vi "9759 RevB Read.vi"(5 "FIFO Indexes.Read":T3, 6 "Device Outputs in":dbl[](array[numeric]), 7 "Settings.PositionCals":T2(array[cluster]), 8 "error in":errorcluster, 9 "dt (sec)":sgl, 11 "FPGA Ref in":T4) -> (0 "error out":errorcluster, 2 "Data":T1, 3 "FPGA Ref out":T4, 4 "Device Outputs out":dbl[](array[numeric]))   [LabVIEW 2015, in "NI 9759 RevB Custom Device.lvlib"]
uses:
  NI 9759 RevB Custom Device.lvlib
  Shared/Types/9759 RevB FPGA Ref.ctl
  <vilib>/Utility/error.llb/Error Cluster From Error Code.vi
  <vilib>/rvi/errors/niLvFpgaAdjustHostInterfaceError.vi
  <vilib>/rvi/interface/nirviReadWriteControl/nirviReadWriteControl.xnode
  NiFpgaLv.dll
  <vilib>/rvi/interface/Simulation/niFpgaSimulationCallBeginRW.vi
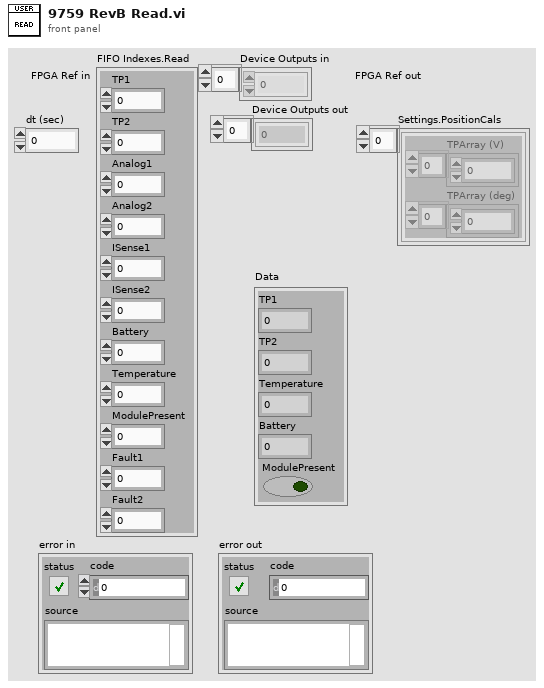
[diagram p1: front panel]
types:
  T1 = cluster{"TP1":sgl, "TP2":sgl, "Temperature":sgl, "Battery":sgl, "ModulePresent":bool}
  T2 = cluster{"TPArray (V)":sgl[], "TPArray (deg)":sgl[]}[]
  T3 = cluster{"TP1":i32, "TP2":i32, "Analog1":i32, "Analog2":i32, "ISense1":i32, "ISense2":i32, "Battery":i32, "Temperature":i32, "ModulePresent":i32, "Fault1":i32, "Fault2":i32}
  T4 = typedef "NI 9759 RevB Custom Device.lvlib/9759 RevB FPGA Ref.ctl" = refnum<k20>
  T5 = cluster{"ModulePresent":bool, "ISense1":i16, "ISense2":i16, "Analog1":i16, "Analog2":i16, "Battery":i16, "Temperature":i16, "Fault1":bool, "Fault2":bool}
  T6 = cluster{"TPArray (V)":sgl[], "TPArray (deg)":sgl[]}
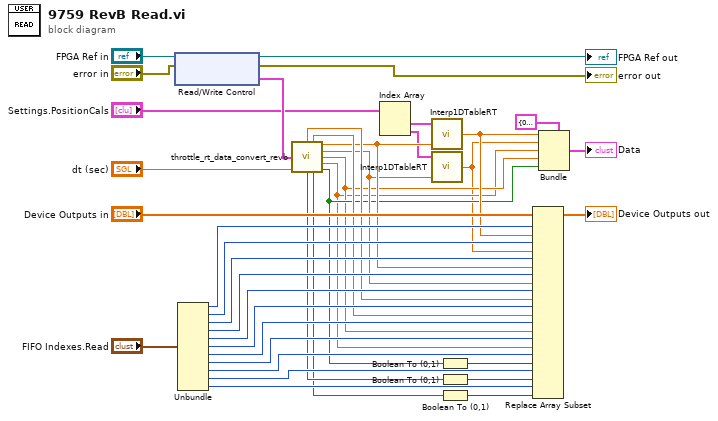
[diagram p0: block diagram]
diagram:
  n1 = xnode "Read/Write Control"("FPGA VI Reference In"="FPGA Ref in", "error in"="error in") -> ("FPGA VI Reference Out"=→"FPGA Ref out":T4, "error out"=→"error out":errorcluster, "ThrottleData"=w37:T5)
  n2 = Unbundle("FIFO Indexes.Read") -> ("TP1"=w33:i32, "TP2"=w32:i32, "Analog1"=w31:i32, "Analog2"=w30:i32, "ISense1"=w29:i32, "ISense2"=w28:i32, "Battery"=w27:i32, "Temperature"=w26:i32, "ModulePresent"=w25:i32, "Fault1"=w24:i32, "Fault2"=w23:i32)
  n3 = call <vilib>:"throttle_rt_data_convert_revb.vi"("ThrottleData"=w37, "dt (sec)"="dt (sec)") -> ("ISense1 (A)"=w16:sgl, "ISense2 (A)"=w17:sgl, "Analog1 (V)"=w13:sgl, "Analog2 (V)"=w12:sgl, "Battery (V)"=w4:sgl, "Temperature (C)"=w3:sgl, "Fault1"=w22:bool, "Fault2"=w21:bool, "ModulePresent"=w5:bool)  [unwired: 5 in]
  n4 = Index Array(array="Settings.PositionCals") -> (element #1=w10:T6, element #2=w9:T6)  [unwired: 2 in]
  n5 = call <vilib>:"Interp1DTableRT.vi"("X"=w13, "1DTable"=w10) -> ("Y"=w6:sgl)  [unwired: 1 in]
  n6 = call <vilib>:"Interp1DTableRT.vi"("X"=w12, "1DTable"=w9) -> ("Y"=w1:sgl)  [unwired: 1 in]
  n7 = Boolean To (0,1)(Boolean=w5) -> (0, 1=w18:i16)
  n8 = Boolean To (0,1)(Boolean=w22) -> (0, 1=w20:i16)
  n9 = Boolean To (0,1)(Boolean=w21) -> (0, 1=w19:i16)
  n10 = Replace Array Subset(array="Device Outputs in", new element #1=w6, index #1=w33, new element #2=w1, index #2=w32, new element #3=w13, index #3=w31, new element #4=w12, index #4=w30, new element #5=w16, index #5=w29, new element #6=w17, index #6=w28, new element #7=w4, index #7=w27, new element #8=w3, index #8=w26, new element #9=w18, index #9=w25, new element #10=w20, index #10=w24, new element #11=w19, index #11=w23) -> (→"Device Outputs out":dbl[])
  n11 = Bundle(cluster=T1 {"TP1"=0.0, "TP2"=0.0, "Temperature"=0.0, "Battery"=0.0, "ModulePresent"=FALSE} ("Data"), "TP1"=w6, "TP2"=w1, "Temperature"=w3, "Battery"=w4, "ModulePresent"=w5) -> (→"Data":T1)
